vi "Set_Active_Device.vi"(8 "error in (no error)":errorcluster, 10 "KinovaDevice":T1) -> (0 "error out":errorcluster)   [LabVIEW 2019]
uses:
  <vilib>/Utility/error.llb/Error Cluster From Error Code.vi
  <vilib>/ErrorRing/Error Ring.xnode
  source/repos/Kinova Labview Interface/Debug/KLInterface.dll
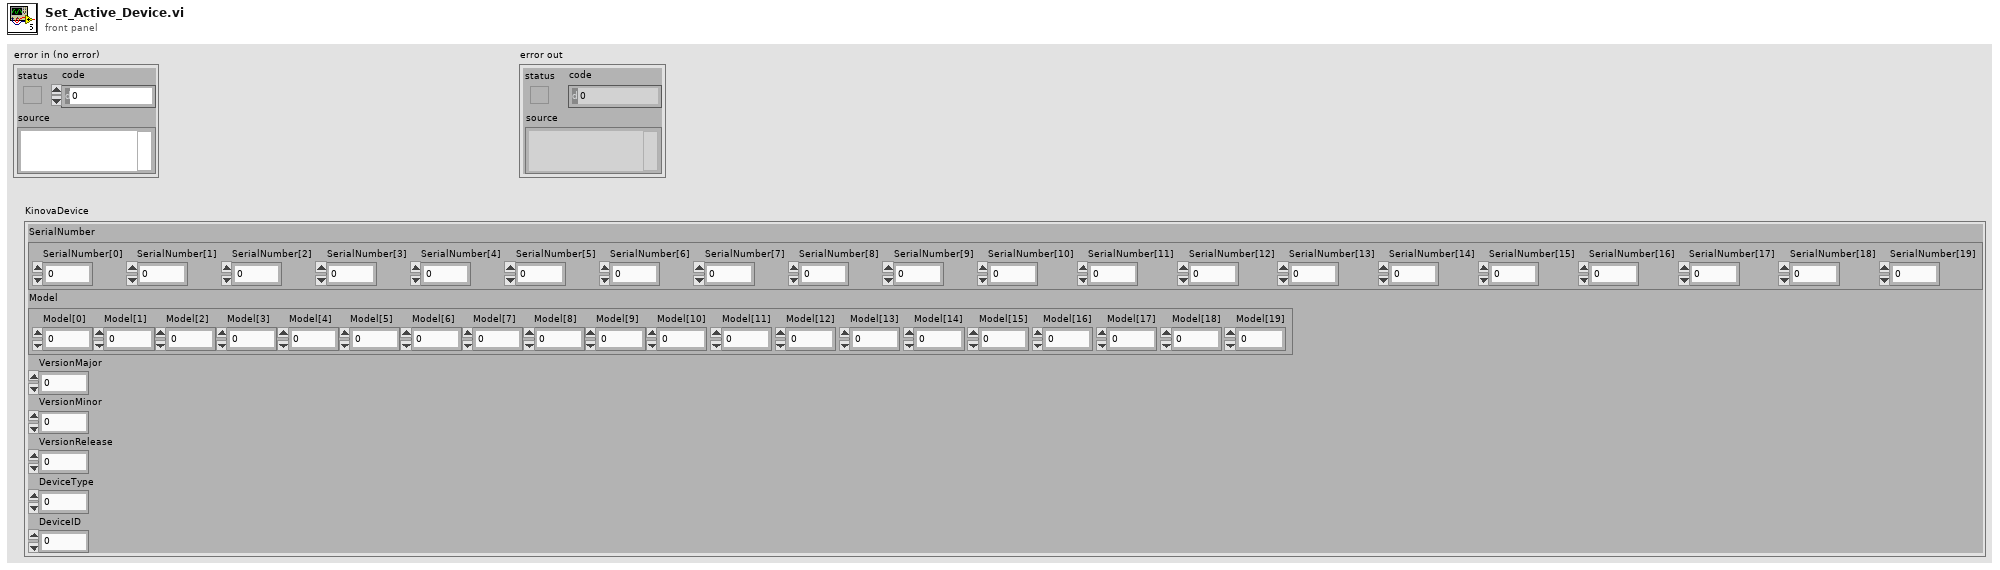
[diagram p1: front panel]
types:
  T1 = cluster{"SerialNumber":cluster{"SerialNumber[0]":u8, "SerialNumber[1]":u8, "SerialNumber[2]":u8, "SerialNumber[3]":u8, "SerialNumber[4]":u8, "SerialNumber[5]":u8, "SerialNumber[6]":u8, "SerialNumber[7]":u8, "SerialNumber[8]":u8, "SerialNumber[9]":u8, "SerialNumber[10]":u8, "SerialNumber[11]":u8, "SerialNumber[12]":u8, "SerialNumber[13]":u8, "SerialNumber[14]":u8, "SerialNumber[15]":u8, "SerialNumber[16]":u8, "SerialNumber[17]":u8, "SerialNumber[18]":u8, "SerialNumber[19]":u8}, "Model":cluster{"Model[0]":u8, "Model[1]":u8, "Model[2]":u8, "Model[3]":u8, "Model[4]":u8, "Model[5]":u8, "Model[6]":u8, "Model[7]":u8, "Model[8]":u8, "Model[9]":u8, "Model[10]":u8, "Model[11]":u8, "Model[12]":u8, "Model[13]":u8, "Model[14]":u8, "Model[15]":u8, "Model[16]":u8, "Model[17]":u8, "Model[18]":u8, "Model[19]":u8}, "VersionMajor":i32, "VersionMinor":i32, "VersionRelease":i32, "DeviceType":i32, "DeviceID":i32}
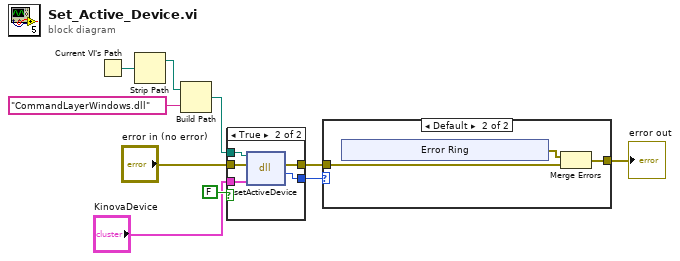
[diagram p0: block diagram]
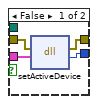
[diagram p2: hidden frame]
diagram:
  n1 = Current VI's Path() -> (path=w9:path)
  n2 = Strip Path(path=w9) -> (stripped path=w8:path)  [unwired: 1 out]
  n3 = Build Path(base path=w8, name or relative path="CommandLayerWindows.dll") -> (appended path=w6:path)
  n4 = case shown="True" FALSE {
    tunnel: w6 -> [_ w19]
    tunnel: "error in (no error)" -> [w14 w18]
    tunnel: [w12 w17] -> w4
    tunnel: [w11 w16] -> w3
    tunnel: "KinovaDevice" -> [w13 w15]
    frame False {
      n5 = dll-call lib="C:/Users/mcjssdcc/source/repos/Kinova Labview Interface/Debug/KLInterface.dll" fn="setActiveDevice"(error in=w14, "device"=w13) -> (error out=w12:errorcluster, "return type"=w11:i32)  [unwired: 3 in, 1 out]
    }
    frame True {
      n6 = dll-call lib="C:/Users/mcjssdcc/source/repos/Kinova Labview Interface/Debug/KLInterface.dll" fn="setActiveDevice"(path in=w19, error in=w18, "device"=w15) -> (error out=w17:errorcluster, "return type"=w16:i32)  [unwired: 2 in, 1 out]
    }
  }
  n7 = case shown="Default" w3 {
    tunnel: [w20 w22] -> w7
    tunnel: w4 -> [w20 w21]
    frame 1 {
    }
    frame Default {
      n8 = xnode "Error Ring"() -> ("error out"=w23:errorcluster)
      n9 = Merge Errors(w23, w21) -> (w22:errorcluster)
    }
  }
  "error out" <- w7
